vi "Status_background.vi"(6 "Display":refnum<vi>, 7 "Action":T2(ring)=enum."¦a¹«¤É°_", 8 "error in (no error)":errorcluster, 9 "Position":cluster{"Row":i32, "Col":i32}, 10 "vi ref":refnum<vi>[][](array[refnum]), 11 "Display Sema":T1) -> (0 "error out":errorcluster)   [LabVIEW 2018]
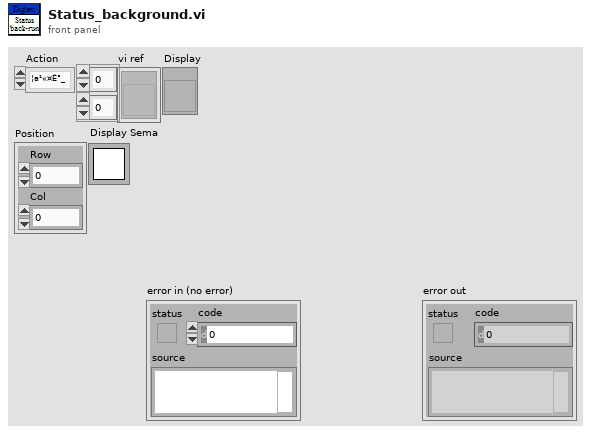
[diagram p1: front panel]
types:
  T1 = typedef "Semaphore RefNum" = refnum<k1>
  T2 = enum16{"ªÅ¬}", "¦a¹«¤É°_", "¦a¹«¤U­°", "¦a¹«³Q¥´", "¥´¿ù¬}"}
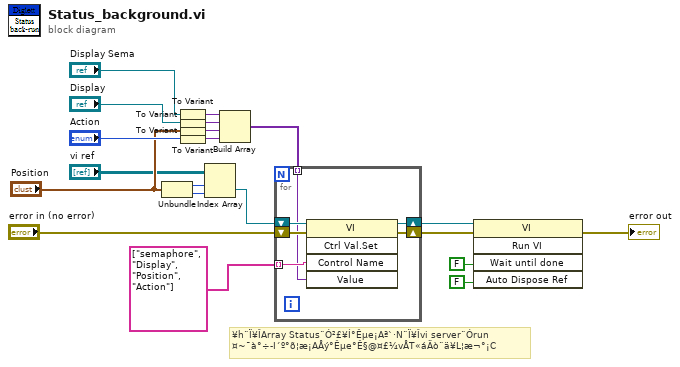
[diagram p0: block diagram]
diagram:
  # "¥h¨Ï¥ÎArray Status¨Ó²£¥Í°Êµe¡Aª`·N¨Ï¥Îvi server¨Órun\n¤~¯à°÷­I´º°õ¦æ¡AÅý°Êµe°Ê§@¤£¼vÅT«áÄò¨ä¥L¦æ¬°¡C"
  n1 = Unbundle("Position") -> ("Row"=w18:i32, "Col"=w17:i32)
  n2 = To Variant(anything="Display Sema") -> (Variant=w12:variant)
  n3 = To Variant(anything="Display") -> (Variant=w13:variant)
  n4 = To Variant(anything="Position") -> (Variant=w14:variant)
  n5 = To Variant(anything="Action") -> (Variant=w15:variant)
  n6 = Index Array(array="vi ref", index (row)=w18, index (col)=w17) -> (element=w20:refnum<vi>)
  n7 = Build Array(w12, w13, w14, w15) -> (w9:variant[])
  n8 = for {
    tunnel: string[] ["semaphore", "Display", "Position", "Action"] -> [w25] mode=indexing
    shift-right: [w24] -> w19
    shift-left: w20 -> [w26]
    shift-right: [w22] -> w10
    shift-left: "error in (no error)" -> [w23]
    tunnel: w9 -> [w21] mode=indexing
    n9 = invoke class="VI" method="Ctrl Val.Set"(reference=w26, error in=w23, "Control Name"=w25, "Value"=w21) -> (reference out=w24:refnum<vi>, error out=w22:errorcluster)  [unwired: 1 in, 3 out]
  }
  n10 = invoke class="VI" method="Run VI"(reference=w19, error in=w10, "Wait until done"=FALSE ("Wait Until Done"), "Auto Dispose Ref"=FALSE ("Auto Dispose Reference")) -> (error out=→"error out":errorcluster)  [unwired: 1 in, 4 out]
